vi "Label Particles.vi"(8 "Color":u32(colorbox)=6618898, 9 "Location":cluster{dbl, dbl}={0.0, 20.0}, 10 "Details":T2, 11 "Image":T1) -> (3 "Image 2":T1)   [LabVIEW 2015]
doc: "Draw text scores near or on the particle."
uses:
  <vilib>/vision/Image Controls.llb/IMAQ Image.ctl
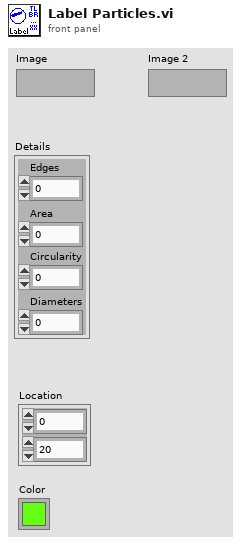
[diagram p1: front panel]
types:
  T1 = typedef "IMAQ Image.ctl" = refnum<image>
  T2 = cluster{"Edges":dbl, "Area":dbl, "Circularity":dbl, "Diameters":dbl}
  T3 = cluster{"Desired Font (Application)":enum16{"User-specified Font", "Application Font", "System Font", "Dialog Font"}, "[User-specified Font]":cluster{"Font Name":string, "Size":i16, "Strikeout?":bool, "Italic?":bool, "Underline?":bool, "Outline?":bool, "Shadow?":bool, "Bold?":bool, "Rotation Angle":dbl}, "Horizontal Alignment":i16, "Vertical Alignment":i16}
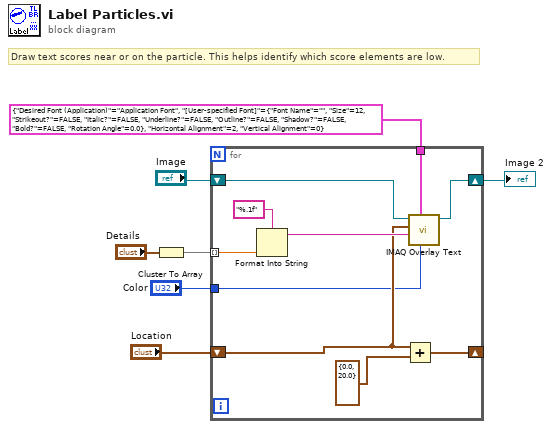
[diagram p0: block diagram]
diagram:
  # "Draw text scores near or on the particle. This helps identify which score elements are low."
  n1 = Cluster To Array(cluster="Details") -> (array=w2:dbl[])
  n2 = for {
    tunnel: T3 {"Desired Font (Application)"=enum."Application Font", "[User-specified Font]"={"Font Name"="", "Size"=12, "Strikeout?"=FALSE, "Italic?"=FALSE, "Underline?"=FALSE, "Outline?"=FALSE, "Shadow?"=FALSE, "Bold?"=FALSE, "Rotation Angle"=0.0}, "Horizontal Alignment"=2, "Vertical Alignment"=0} ("Font, Size & Style") -> [w17]
    tunnel: w2 -> [w9] mode=indexing
    shift-right: [w13] -> _
    shift-left: "Location" -> [w11]
    shift-right: [w14] -> w5
    shift-left: "Image" -> [w15]
    tunnel: "Color" -> [w8]
    n3 = Format Into String(format string="%.1f", w9) -> (resulting string=w16:string)  [unwired: 2 in, 1 out]
    n4 = Add(x=cluster{dbl, dbl} {0.0, 20.0} ("x+y"), y=w11) -> (x+y=w13:cluster{dbl, dbl})
    n5 = call "IMAQ Overlay Text"("Text Color (black)"=w8, "Font, Size & Style"=w17, "String"=w16, "Origin"=w11, "Image"=w15) -> ("Image Out"=w14:T1)  [unwired: 5 in, 1 out]
  }
  "Image 2" <- w5
